vi "TDMS Convert.vi"() -> ()   [LabVIEW 2014]
uses:
  <vilib>/Utility/error.llb/DialogType.ctl
  <vilib>/Utility/file.llb/Write To Spreadsheet File (string).vi
panel:
  in  "Path":path
  out "Exit":bool
  out "Stop":bool
  out "Converting...":u64(slide) scale=0.0..100.0
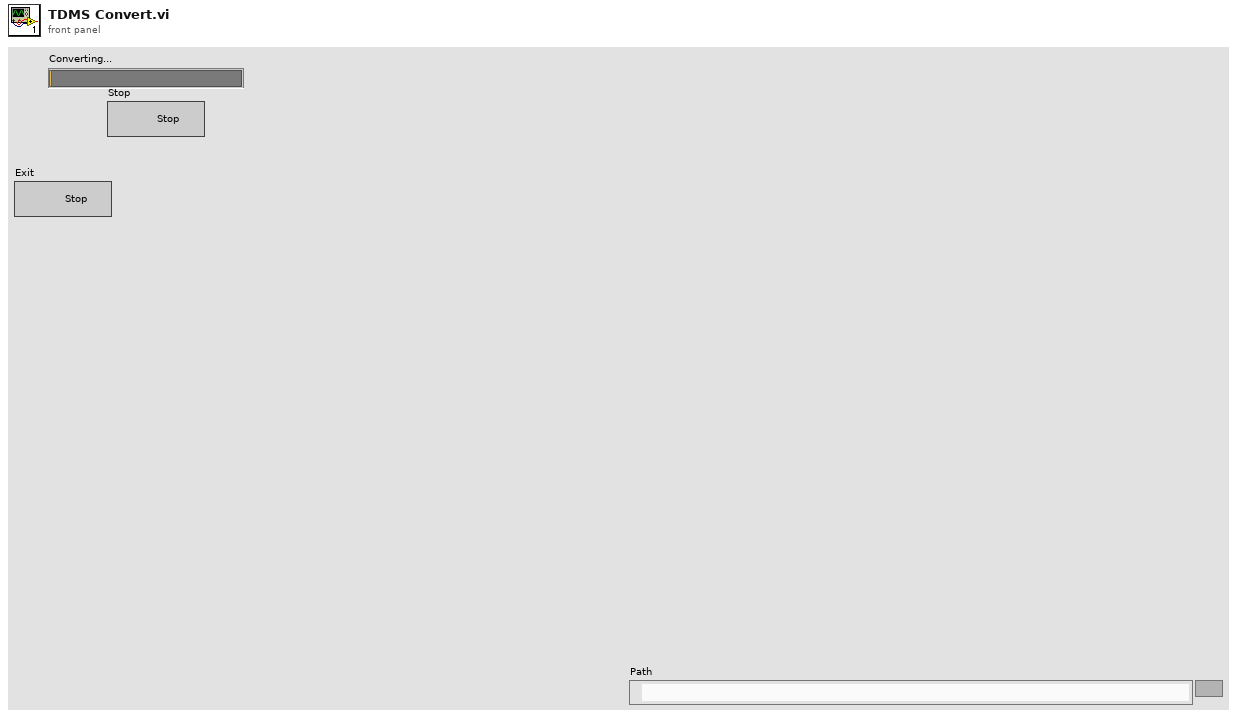
[diagram p1: front panel]
types:
  T1 = typedef "DialogType.ctl" = u16
  T2 = enum16{"open", "open or create", "create or replace", "create", "open (read-only)"}
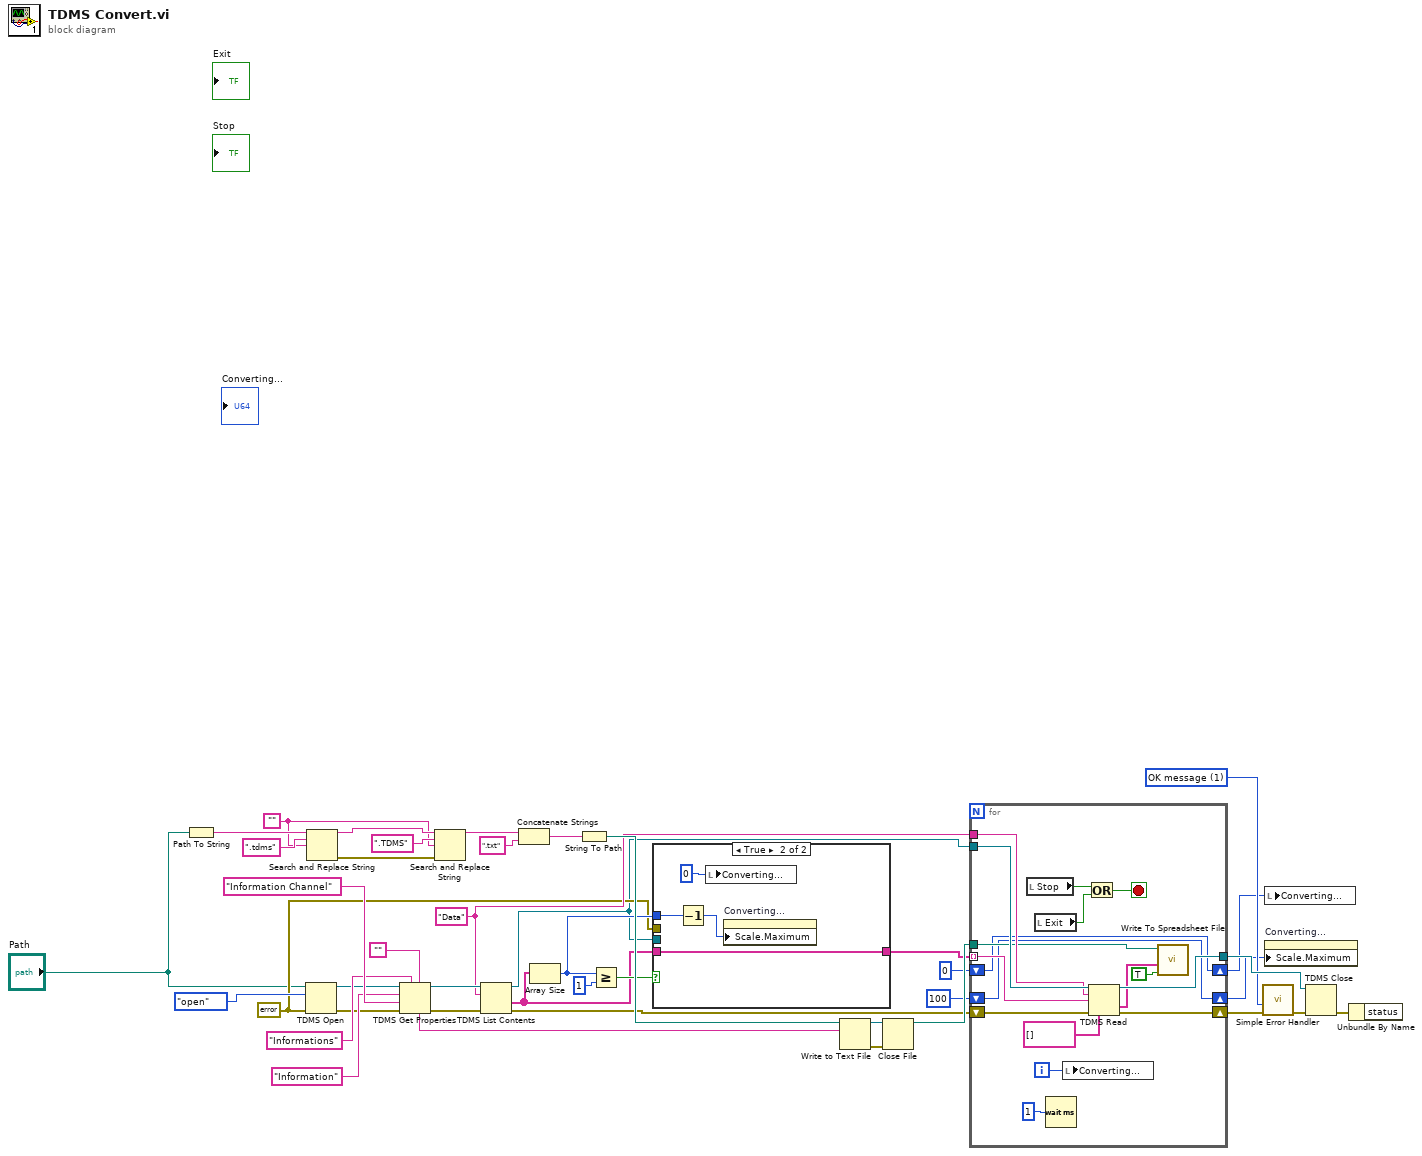
[diagram p0: block diagram]
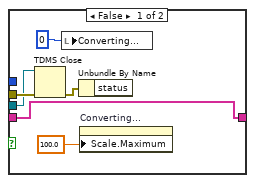
[diagram p2: hidden frame]
diagram:
  w18 = T1 1 items=["no dialog", "OK message", "continue or stop message", "OK message + warnings", "continue/stop + warnings"] ("type of dialog (OK msg:1)")
  w8 = errorcluster {"status"=FALSE, "code"=0, "source"=""} ("error in (no error)")
  w35 = ""
  w30 = "Data" ("group name")
  n1 = Path To String(path="Path") -> (string=w39:string)
  n2 = TDMS Open(8:w8, 10:T2."open" ("operation (0:open)"), 11:"Path") -> (0:w20:errorcluster, 3:w12:refnum<k34>)  [unwired: 4 in]
  n3 = Search and Replace String(input string=w39, search string=".tdms", replace string=w35) -> (result string=w37:string, error out=w34:errorcluster)  [unwired: 5 in, 2 out]
  n4 = TDMS Get Properties(5:"", 7:"Informations" ("property names"), 8:w20, 9:"Information Channel" ("channel name"), 10:"Information" ("group name"), 11:w12) -> (0:w28:errorcluster, 3:w31:refnum<k34>, 4:w32:string)  [unwired: 3 out]
  n5 = Search and Replace String(input string=w37, search string=".TDMS", replace string=w35, error in=w34) -> (result string=w22:string)  [unwired: 4 in, 3 out]
  n6 = TDMS List Contents(4:w28, 6:w30, 7:w31) -> (0:w14:errorcluster, 1:w6:string[], 3:w7:refnum<k34>)  [unwired: 1 out]
  n7 = Concatenate Strings(w22, ".txt" ("string")) -> (w23:string)
  n8 = Array Size(array=w6) -> (size(s)=w11:i32)
  n9 = String To Path(string=w23) -> (path=w33:path)
  n10 = Greater Or Equal?(x=w11, y=1) -> (x >= y?=w9:bool)
  n11 = case shown="True" w9 {
    tunnel: w11 -> [_ w51]
    tunnel: w8 -> [w47 _]
    tunnel: w7 -> [w46 _]
    tunnel: [w44 w50] -> w5
    tunnel: w6 -> [w44 w50]
    frame False {
      n12 = TDMS Close(8:w47, 11:w46) -> (0:w48:errorcluster)  [unwired: 1 out]
      n13 = local write "Converting..."(u64 0 ("Converting...")) -> ()
      n14 = Unbundle By Name(w48) -> ()  [unwired: 1 out]
      n15 = property on="Converting..." class="Slide (strict)"("Scale.Maximum"=100.0 ("Scale.Range:Maximum")) -> ()  [unwired: 2 in, 2 out]
    }
    frame True {
      n16 = Decrement(x=w51) -> (x-1=w52:i32)
      n17 = local write "Converting..."(u64 0 ("Converting...")) -> ()
      n18 = property on="Converting..." class="Slide (strict)"("Scale.Maximum"=w52) -> ()  [unwired: 2 in, 2 out]
    }
  }
  n19 = Write to Text File(file (use dialog)=w33, text=w32) -> (refnum out=w27:refnum<file>, error out=w26:errorcluster)  [unwired: 2 in, 1 out]
  n20 = Close File(refnum=w27, error in=w26) -> (path=w25:path)  [unwired: 1 out]
  n21 = for {
    tunnel: w30 -> [w68]
    tunnel: w7 -> [w69]
    shift-right: [w66] -> w16
    shift-left: w14 -> [w67]
    tunnel: w5 -> [w65] mode=indexing
    tunnel: [w63] -> w24
    tunnel: w25 -> [w62]
    shift-right: [w54] -> w4
    shift-left: u8 100 ("Converting...") -> [w54]
    shift-right: [w53] -> w17
    shift-left: u8 0 ("Converting...") -> [w53]
    i -> [w59]
    stop <- w56 stop-if-true
    n22 = local read "Stop"() -> (w58:bool)
    n23 = local read "Exit"() -> (w57:bool)
    n24 = Wait (ms)(milliseconds to wait=u32 1) -> ()  [unwired: 1 out]
    n25 = local write "Converting..."(w59) -> ()
    n26 = Or(x=w58, y=w57) -> (x .or. y?=w56:bool)
    n27 = TDMS Read(0:w69, 5:w68, 7:w65, 11:w67, 12:string[] []) -> (4:w63:refnum<k34>, 10:w60:string[], 15:w66:errorcluster)  [unwired: 3 in, 3 out]
    n28 = call-poly <vilib>:"Write To Spreadsheet File.vi"("append to file? (new file:F)"=TRUE, "1D data"=w60, "file path (dialog if empty)"=w62) -> ()  [unwired: 5 in, 1 out]
  }
  n29 = call <vilib>:"Simple Error Handler.vi"("type of dialog (OK msg:1)"=w18, "error in (no error)"=w16) -> ("error out"=w13:errorcluster)  [unwired: 3 in, 4 out]
  n30 = local write "Converting..."(w17) -> ()
  n31 = property on="Converting..." class="Slide (strict)"("Scale.Maximum"=w4) -> ()  [unwired: 2 in, 2 out]
  n32 = TDMS Close(8:w13, 11:w24) -> (0:w15:errorcluster)  [unwired: 1 out]
  n33 = Unbundle By Name(w15) -> ()  [unwired: 1 out]
